vi "RP Transceiver Test.vi"() -> ()   [LabVIEW 2024]
uses:
  RP Transceiver.lvclass
  Receiver format.ctl
panel:
  in  "Step":dbl
  in  "End":dbl
  in  "Start":dbl
  in  "Server address":string="192.168.1.100"
  in  "Averaging time":dbl format="%#_6p"
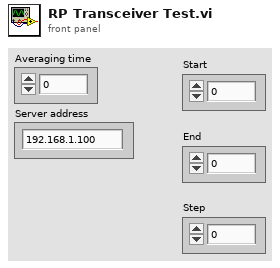
[diagram p1: front panel]
types:
  T1 = typedef "Receiver format.ctl" = enum16{"X-Y-F", "F-X-Y", "X-Y", "X"}
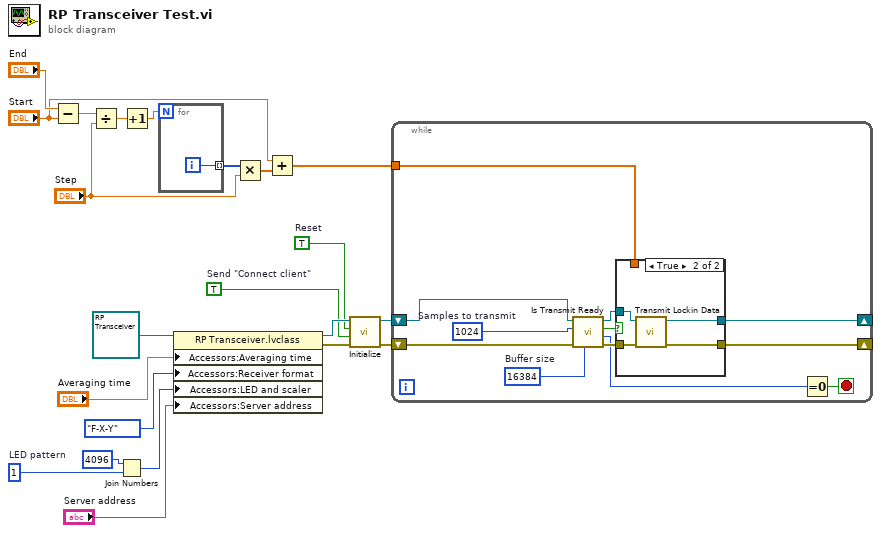
[diagram p0: block diagram]
diagram:
  w12 = TRUE  # Send "Connect client"
  w13 = TRUE  # Reset
  w17 = i16 1  # LED pattern
  n1 = Subtract(x="End", y="Start") -> (x-y=w8:dbl)
  n2 = Divide(x=w8, y="Step") -> (x/y=w7:dbl)
  n3 = Join Numbers(hi=i16 4096, lo=w17) -> ((hi.lo)=w19:u32)
  n4 = Increment(x=w7) -> (x+1=w6:dbl)
  n5 = for {
    N: w6 -> [_]
    tunnel: [w23] -> w5 mode=indexing
    i -> [w23]
  }
  n6 = property class="RP Transceiver.lvclass"(reference=refnum<class "RP Transceiver.lvclass"> refnum ("RP Transceiver.lvclass"), "Accessors:Averaging time"="Averaging time", "Accessors:Receiver format"=Receiver_format."F-X-Y" ("Receiver format"), "Accessors:LED and scaler"=w19, "Accessors:Server address"="Server address") -> (reference out=w15:refnum<class "RP Transceiver.lvclass">, error out=w14:errorcluster)  [unwired: 1 in]
  n7 = Multiply(x=w5, y="Step") -> (x*y=w3:dbl[])
  n8 = Add(x="Start", y=w3) -> (x+y=w1:dbl[])
  n9 = call-dynamic "Initialize.vi"("error in (no error)"=w14, "Send \"Connect client\""=w12, "Reset"=w13, "RP Transceiver in"=w15) -> ("error out"=w10:errorcluster, "RP Transceiver out"=w11:refnum<class "RP Transceiver.lvclass">)  [unwired: 6 in]
  n10 = while {
    shift-right: [w26] -> _
    shift-left: w11 -> [w32]
    shift-right: [w27] -> _
    shift-left: w10 -> [w35]
    tunnel: w1 -> [w28]
    stop <- w24 stop-if-true
    w33 = 1024  # Samples to transmit
    w34 = 16384  # Buffer size
    n11 = call-dynamic "Is Transmit Ready.vi"("Buffer size"=w34, "error in (no error)"=w35, "Samples to transmit"=w33, "RP Instrument in"=w32) -> ("error out"=w30:errorcluster, "Unused buffer"=w25:i32, "Transmit Ready"=w31:bool, "RP Instrument out"=w29:refnum<class "RP Transceiver.lvclass">)  [unwired: 4 in]
    n12 = case shown="True" w31 {
      tunnel: w30 -> [w37 w41]
      tunnel: w29 -> [w36 w40]
      tunnel: w28 -> [_ _]
      tunnel: [w37 w39] -> w27
      tunnel: [w36 w38] -> w26
      frame False {
      }
      frame True {
        n13 = call-dynamic "Transmit Lockin Data.vi"("error in (no error)"=w41, "RP Transceiver in"=w40) -> ("error out"=w39:errorcluster, "RP Transceiver out"=w38:refnum<class "RP Transceiver.lvclass">)  [unwired: 7 in, 1 out]
      }
    }
    n14 = Equal To 0?(x=w25) -> (x = 0?=w24:bool)
  }
